vi "SR430.get bin data.vi"(0 "i ref in":refnum<vi>, 5 "error in (no error)":errorcluster) -> (14 "i ref out":refnum<vi>, 16 "Output Waveform":waveform(dbl), 19 "error out":errorcluster)   [LabVIEW 2014, in "SR430.lvlib"]
doc: "gets the data in binary format from the SR430. The data format is a waveform."
uses:
  SR430.lvlib
  CSCore/CSApplicationBaseClasses/MCSBase/MCSBase.directionType.ctl
  CSCore/CSApplicationBaseClasses/MCSBase/MCSBase.serviceType.ctl
  CSCore/CSSystem/CoreDefs/CoreDefs.error_type.ctl
  CSinstr.lib/Sr430/SR430Driver.lvlib
  CSCore/CSSystem/CoreLib/CoreLib.lvlib
  CSCore/CSApplicationBaseClasses/MCSBase/MCSBase.lvlib
  CSlibraries/UtilityLib/UtilityLib.lvlib
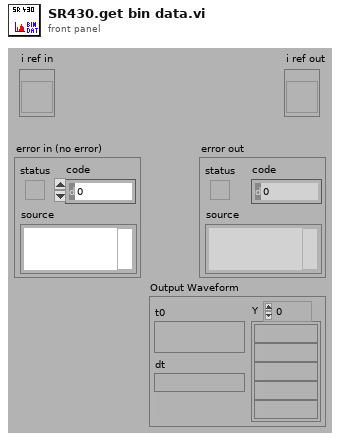
[diagram p1: front panel]
types:
  T1 = typedef "MCSBase.lvlib/MCSBase.serviceType.ctl" = enum16{"counts", "totalCounts", "binWidth", "nOfBins", "nOfRecords", "status", "discrLevel", "discrSlope", "triggerLevel", "triggerSlope"}
  T2 = typedef "CoreDefs.error_type.ctl" = enum16{"no error", "can't load process", "can't unload process", "process does not exist", "can't install process", "can't remove process", "unknown function", "time out", "can't execute function", "duplicate queue name", "super not found", "caller queue invalid", "can't ping process", "unknown error", "VISA Error", "VISA timeout", "GPIB timeout", "GPIB error", "communication error", "data type mismatch", "can't read data from OPC server", "can't write data to OPC server", "OET error", "function not implemented", "process already exists", "invalid Shared Variable name", "error writing Shared Variable", "error reading Shared Variable", "invalid client name", "corrupt database", "unknown class", "call not authorized", "parameter out of range", "OET timeout: can't get data to modify", "invalid queue name", "requested operation incompatible with current state", "event undefined", "event disabled", "state undefined", "caller is not a friend", "EventBuilder: bad eventID", "EventBuilder: no DAQ devices", "a thread must not stop itself", "UNUSED ELEMENT4", "DiscArchiver: eventData incomplete", "DiscArchiver: eventData does not belong to run", "DiscArchiver: can't open file", "DiscArchiver: can't write to file", "DiscArchiver: available disc space low", "can't acquire semaphore", "error reading data from database", "notifier object is not existing", "can't register process", "can't unregister process", "illegal event type", "object disabled", "object already exists", "can't change state", "Instrument not found", "no connection to remote node", "invalid reference", "N/A", "UNUSED ELEMENT 1", "element not found", "illegal TCP/IP connection detected", "object does not exist", "invalid access ID", "unknown CS system", "invalid privilige", "unsupported data type", "unsupported server type", "IO server already exists", "Shared Variable already exists"}
  T3 = typedef "MCSBase.lvlib/MCSBase.directionType.ctl" = enum16{"unknown", "update actual value", "update nominal value", "update both"}
  T4 = typedef "SR430Driver.lvlib/SR430_VISA Control.ctl" = cluster{"VISA resource name":refnum<visa-resource-name>}
  T5 = typedef "MCSBase.lvlib/MCSBase.i attribute.ctl" = cluster{"actValues":T6, "nomValues":T6}
  T6 = typedef "MCSBase.lvlib/MCSBase.parameters.ctl" = cluster{"counts":i32, "totalCounts":i32, "status":i32, "binWidth [us]":dbl, "nOfBins":i32, "nOfRecords":i32, "discLevel [V]":dbl, "discSlope":bool, "triggerLevel [V]":dbl, "triggerSlope":bool, "serviceIDs":cluster{"countslID":i32, "totalCountsID":i32, "binWidthID":i32, "nOfBinsID":i32, "nOfRecordsID":i32, "statusID":i32, "discLevelID":i32, "discSlopeID":i32, "triggerLevelID":i32, "triggerSlopeID":i32}}
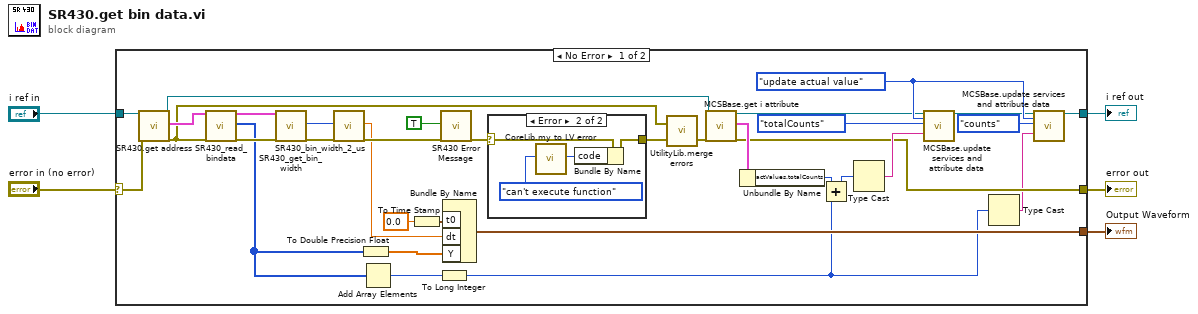
[diagram p0: block diagram]
diagram:
  n1 = case shown="No Error" "error in (no error)" {
    selector: "error in (no error)" -> [w23 w45]
    tunnel: "i ref in" -> [w39 w46]
    tunnel: [w8 w45] -> w4
    tunnel: [w7 w46] -> w3
    tunnel: [w36 _] -> w2
    frame No Error {
      w21 = MCSBase.directionType."update actual value" ("direction")
      n2 = call "SR430.get address.vi"("i ref in"=w39, "error in (no error)"=w23) -> ("i ref out"=w12:refnum<vi>, "address"=w38:T4, "error out"=w37:errorcluster)  [unwired: 15 in]
      n3 = call "SR430_read_bindata.vi"("address"=w38, "error in (no error)"=w37) -> ("address out"=w32:T4, "Data"=w11:u16[], "error out"=w33:errorcluster)  [unwired: 14 in, 1 out]
      n4 = call "SR430_get_bin_width.vi"("address"=w32, "error in (no error)"=w33) -> ("bin width"=w30:i32, "error out"=w31:errorcluster)  [unwired: 15 in, 1 out]
      n5 = call "SR430_bin_width_2_us.vi"("bin width"=w30, "error in (no error)"=w31) -> ("binWidth [us]"=w28:dbl, "error out"=w29:errorcluster)  [unwired: 15 in, 1 out]
      n6 = To Double Precision Float(number=w11) -> (double precision float=w34:dbl[])
      n7 = Add Array Elements(numeric array=w11) -> (sum=w10:u16)
      n8 = To Time Stamp(1:0.0 ("t0")) -> (0:w24:timestamp)
      n9 = To Long Integer(number=w10) -> (32bit integer=w9:i32)
      n10 = call "SR430 Error Message.vi"("addMessageToSource"=TRUE ("add message to source"), "error in (no error)"=w29) -> ("error out"=w35:errorcluster)  [unwired: 14 in, 3 out]
      n11 = Bundle By Name ("Build Waveform")("t0"=w24, "dt"=w28, "Y"=w34) -> (w36:waveform(dbl))  [unwired: 1 in]
      n12 = case shown="Error" w35 {
        selector: w35 -> [w40 w44]
        tunnel: [w40 w41] -> w25
        frame No Error {
        }
        frame Error {
          n13 = call "CoreLib.my to LV error.vi"("ErrorTypes"=CoreDefs.error_type."can't execute function") -> ("LV error code"=w43:i32)  [unwired: 17 in, 1 out]
          n14 = Bundle By Name(cluster=w44, "code"=w43) -> (w41:errorcluster)
        }
      }
      n15 = call "UtilityLib.merge errors.vi"("error2 (no error)"=w25, "error1 (no error)"=w37) -> ("error out"=w13:errorcluster)
      n16 = call "MCSBase.get i attribute.vi"("i ref in"=w12, "error in (no error)"=w13) -> ("i ref out"=w16:refnum<vi>, "i attribute"=w14:T5, "error out"=w8:errorcluster)  [unwired: 15 in]
      n17 = Unbundle By Name(w14) -> ("actValues.totalCounts"=w15:i32)
      n18 = Add(x=w15, y=w9) -> (x+y=w18:i32)
      n19 = Type Cast(x=w18) -> (*(type *) &x=w19:string)  [unwired: 1 in]
      n20 = call "MCSBase.update services and attribute data.vi"("i ref in"=w16, "direction"=w21, "service"=MCSBase.serviceType."totalCounts", "value"=w19) -> ("i ref out"=w20:refnum<vi>)  [unwired: 13 in, 2 out]
      n21 = Type Cast(x=w9) -> (*(type *) &x=w6:string)  [unwired: 1 in]
      n22 = call "MCSBase.update services and attribute data.vi"("i ref in"=w20, "direction"=w21, "service"=MCSBase.serviceType."counts", "value"=w6) -> ("i ref out"=w7:refnum<vi>)  [unwired: 13 in, 2 out]
    }
    frame Error {
    }
  }
  "error out" <- w4
  "i ref out" <- w3
  "Output Waveform" <- w2
